vi "FirePneumaticHandler.vi"(8 "error in (no error)":errorcluster, 9 "cFirePneumatic":bool, 10 "cLauncherWheel":bool, 11 "cQuickShoot":bool) -> (0 "error out":errorcluster)   [LabVIEW 2012]
doc: "Takes the button value for FirePneumatic and determines if it has changed. If it has, enqueues an instruction."
uses:
  QueueInstruction.ctl
  SubsystemEnum.ctl
  ActionEnum.ctl
  Robot Global Data.vi
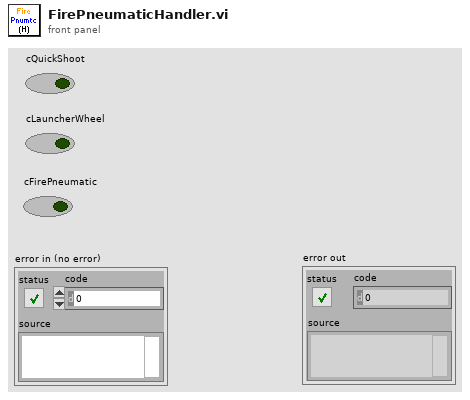
[diagram p1: front panel]
types:
  T1 = typedef "ActionEnum.ctl" = enum16{"Init", "SetValue"}
  T2 = typedef "SubsystemEnum.ctl" = enum16{"TankDrive", "FirePneumatic", "Climber", "ClimbWeight", "ShooterAngle"}
  T3 = typedef "QueueInstruction.ctl" = cluster{"Data":variant, "Subsystem":T2, "Action":T1}
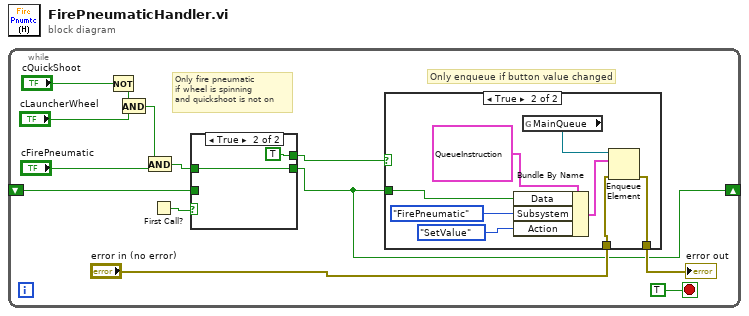
[diagram p0: block diagram]
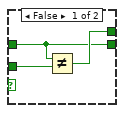
[diagram p3: hidden frame]
diagram:
  n1 = while {
    shift-right: [w1] -> _
    shift-left: _ -> [w11]
    stop <- TRUE stop-if-true
    # "Only enqueue if button value changed"
    # "Only fire pneumatic\nif wheel is spinning\nand quickshoot is not on"
    n2 = Not(x="cQuickShoot") -> (.not. x?=w10:bool)
    n3 = And(x=w10, y="cLauncherWheel") -> (x .and. y?=w9:bool)
    n4 = And(x=w9, y="cFirePneumatic") -> (x .and. y?=w5:bool)
    n5 = First Call?() -> (First Call?: T/F=w12:bool)
    n6 = case shown="True" w12 {
      tunnel: w11 -> [w24 _]
      tunnel: [w25 TRUE] -> w4
      tunnel: w5 -> [w23 w27]
      tunnel: [w23 w27] -> w1
      frame False {
        n7 = Not Equal?(x=w23, y=w24) -> (x != y?=w25:bool)
      }
      frame True {
      }
    }
    n8 = case shown="True" w4 {
      tunnel: w1 -> [_ w20]
      tunnel: "error in (no error)" -> [w14 w16]
      tunnel: [w14 w15] -> w2
      frame False {
      }
      frame True {
        n9 = Bundle By Name(cluster=T3 {"Data"=variant, "Subsystem"=enum."TankDrive", "Action"=enum."Init"} ("QueueInstruction"), "Data"=w20, "Subsystem"=SubsystemEnum."FirePneumatic", "Action"=ActionEnum."SetValue") -> (w17:T3)
        n10 = global read "Robot Global Data.vi" "MainQueue"() -> (w22:refnum<queue>)
        n11 = Enqueue Element(queue=w22, element=w17, error in (no error)=w16) -> (error out=w15:errorcluster)  [unwired: 1 in, 2 out]
      }
    }
    "error out" <- w2
  }
